vi "Generate Simulated Data.vi"(7 "Type de mode":bool, 8 "error in (no error)":T2 caption="entrée d'erreur (pas d'erreur)", 9 "Péri":tag="Dev1", 10 "Longueur d'onde":dbl, 11 "Type de signal":T1) -> (0 "error out":T2 caption="sortie d'erreur", 2 "Données du graphe":waveform(dbl)[](array[waveform]))   [LabVIEW 2018, in "Acquisition.lvlib"]
doc: "Génère des exemples de waveforms en fonction du type de signal dans l'entrée Configuration du matériel."
uses:
  Acquisition.lvlib
  <vilib>/Analysis/NI_AALBase.lvlib
  Signal Type.ctl
panel:
  out "Graphe déroulant":dynamicdata(graph)
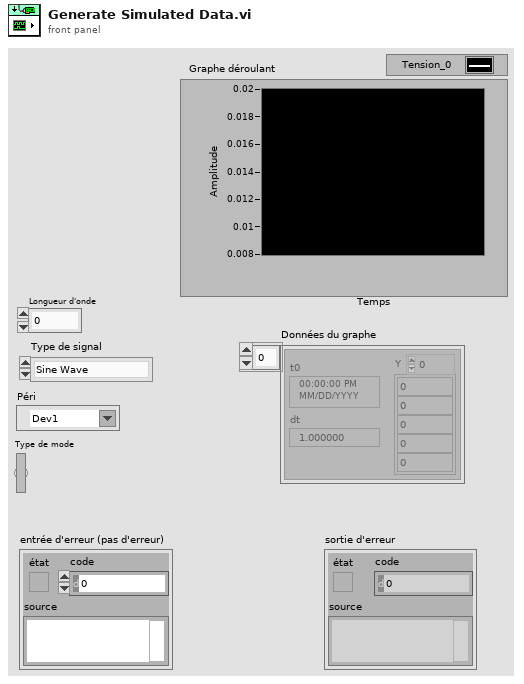
[diagram p1: front panel]
types:
  T1 = typedef "Acquisition.lvlib/Signal Type.ctl" = enum16{"Sine Wave", "Square with Noise", "Signal triangulaire", "Simulation DAQ"}
  T2 = cluster{"état":bool, "code":i32, "source":string}
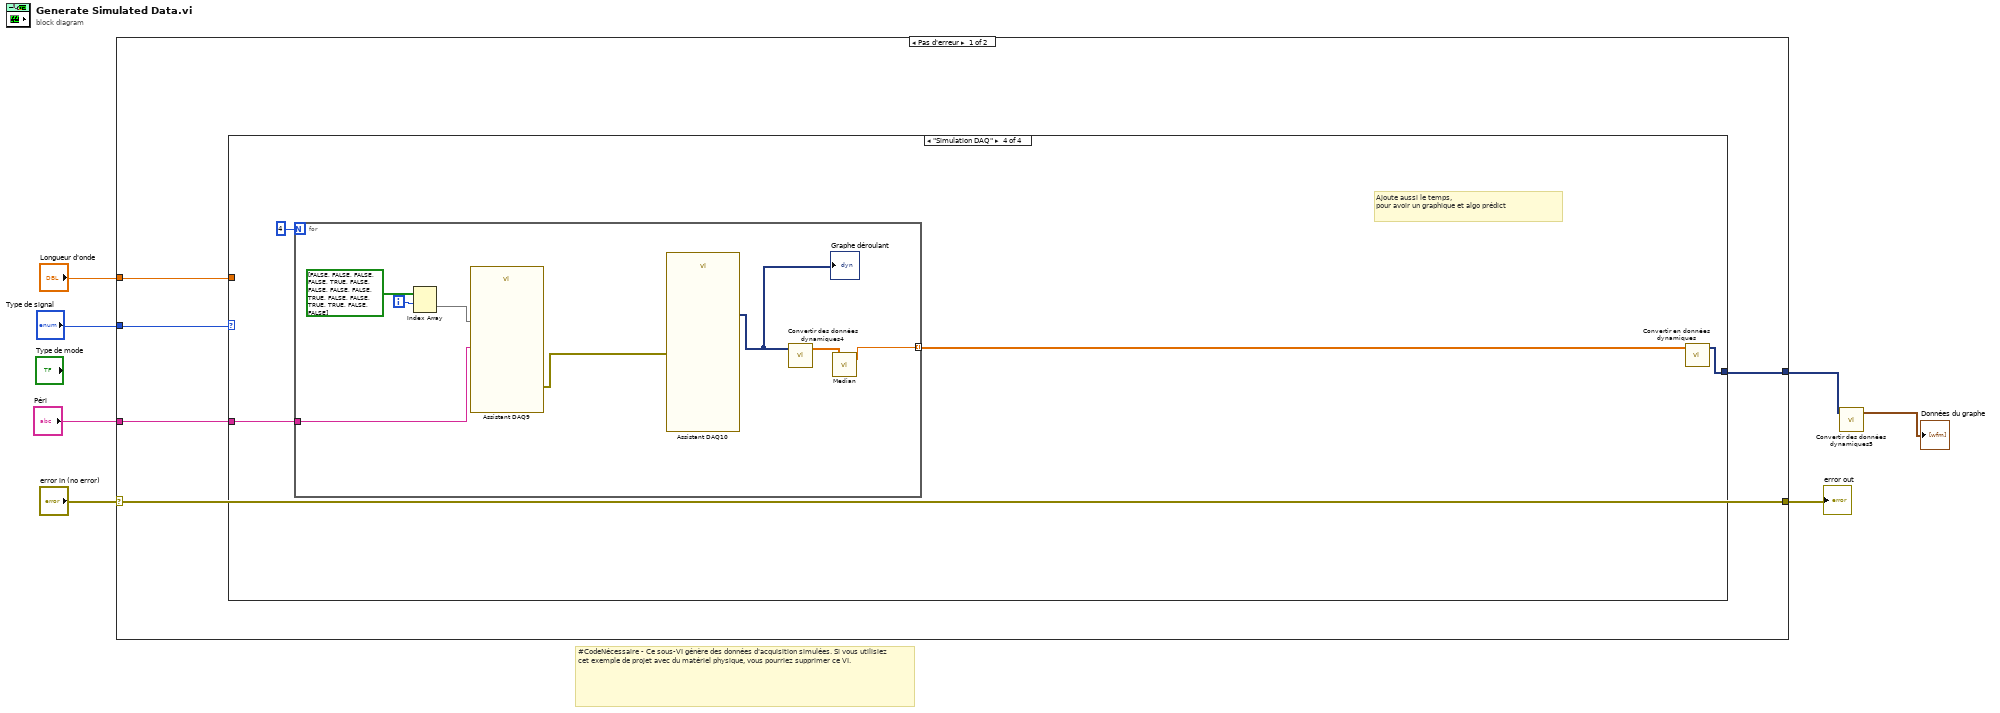
[diagram p0: block diagram]
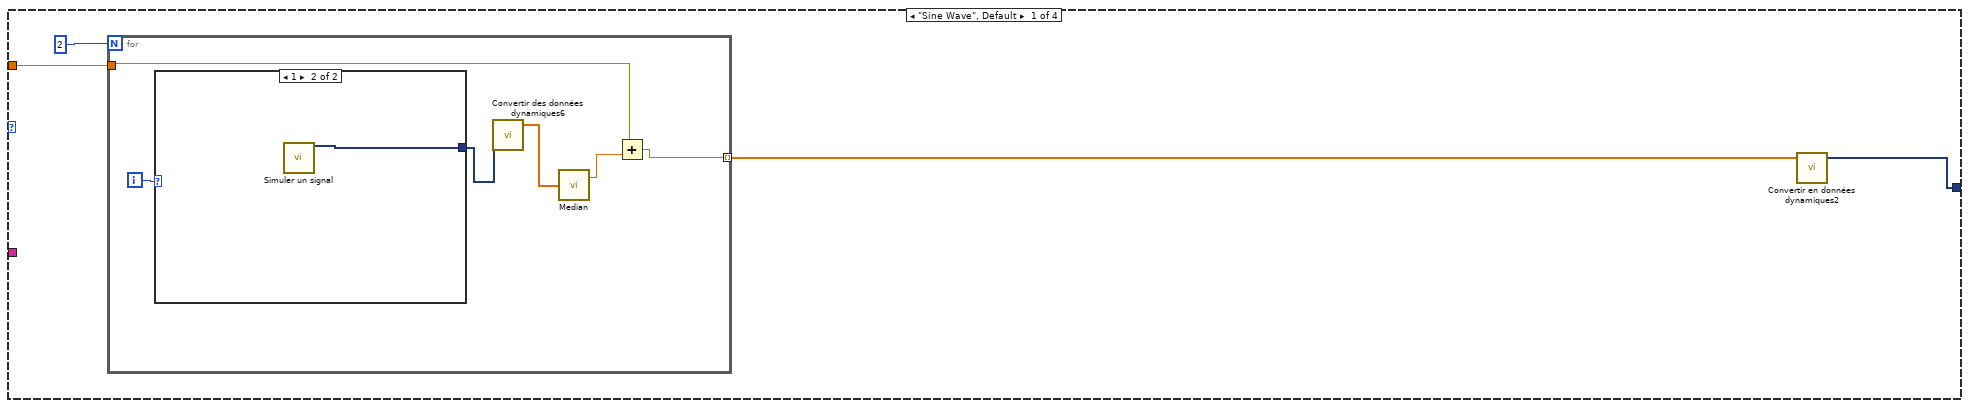
[diagram p2: hidden frame]
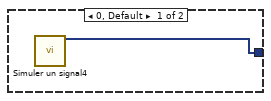
[diagram p3: hidden frame]
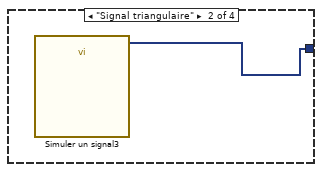
[diagram p4: hidden frame]
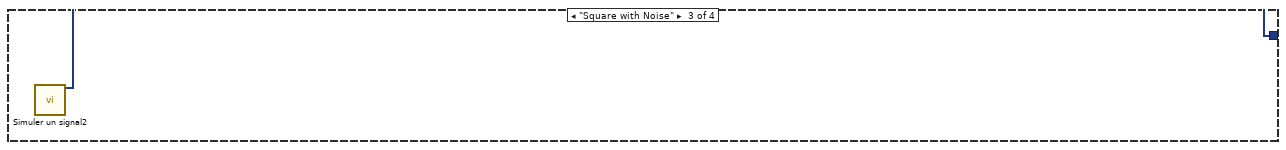
[diagram p5: hidden frame]
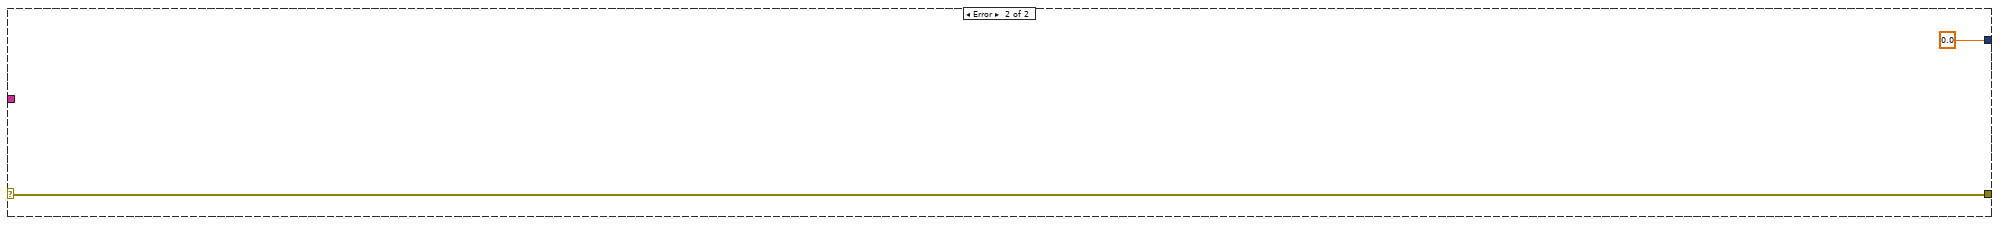
[diagram p6: hidden frame]
diagram:
  # "#CodeNécessaire - Ce sous-VI génère des données d'acquisition simulées. Si vous utilisiez cet exemple de projet avec du matériel physique, vous pourriez supprimer ce VI."
  n1 = case shown="Pas d'erreur" "error in (no error)" {
    selector: "error in (no error)" -> [w12 w40]
    tunnel: [w12 w40] -> w6
    tunnel: "Type de signal" -> [w11 _]
    tunnel: [w10 0.0] -> w3
    tunnel: "Longueur d'onde" -> [w9 _]
    tunnel: "Péri" -> [w8 _]
    frame No Error {
      n2 = case shown="\"Simulation DAQ\"" w11 {
        tunnel: [w15 w25 w26 w29] -> w10
        tunnel: w9 -> [w13 _ _ _]
        tunnel: w8 -> [_ _ _ w27]
        frame "Sine Wave", Default {
          n3 = for {
            N: 2 -> [_]
            tunnel: [w18] -> w14 mode=indexing
            tunnel: w13 -> [w17]
            i -> [w22]
            n4 = case shown="1" w22 {
              tunnel: [w23 w24] -> w21
              frame 0, Default {
                n5 = call "Simuler un signal4"() -> ("CC"=w23:dynamicdata)  [unwired: 14 in, 1 out]
              }
              frame 1 {
                n6 = call "Simuler un signal"() -> ("Sinus avec Bruit uniforme"=w24:dynamicdata)  [unwired: 14 in, 1 out]
              }
            }
            n7 = call "Convertir des données dynamiques6"("Dynamic Data Type"=w21) -> ("Array"=w20:dbl[])  [unwired: 3 in]
            n8 = call <vilib>:"Median.vi"("X"=w20) -> ("median"=w19:dbl)  [unwired: 1 out]
            n9 = Add(x=w17, y=w19) -> (x+y=w18:dbl)
          }
          n10 = call "Convertir en données dynamiques2"("Array"=w14) -> ("Dynamic Data Type"=w15:dynamicdata)  [unwired: 3 in]
        }
        frame "Signal triangulaire" {
          n11 = call "Simuler un signal3"() -> ("Triangle"=w25:dynamicdata)  [unwired: 14 in, 1 out]
        }
        frame "Square with Noise" {
          n12 = call "Simuler un signal2"() -> ("Square with Gaussian Noise"=w26:dynamicdata)  [unwired: 14 in, 1 out]
        }
        frame "Simulation DAQ" {
          # "Ajoute aussi le temps,\npour avoir un graphique et algo prédict"
          n13 = for {
            N: 4 -> [_]
            tunnel: [w38] -> w28 mode=indexing
            tunnel: w27 -> [w31]
            i -> [w33]
            n14 = Index Array(array=bool[][] [[FALSE, FALSE, FALSE, FALSE], [TRUE, FALSE, FALSE, FALSE], [FALSE, TRUE, FALSE, FALSE], [TRUE, TRUE, FALSE, FALSE]], index (row)=w33) -> (element=w32:bool[])  [unwired: 1 in]
            n15 = call "Assistant DAQ9"("data"=w32, "nom du périphérique"=w31) -> ("error out"=w36:errorcluster)  [unwired: 16 in, 1 out]
            n16 = call "Assistant DAQ10"("error in"=w36) -> ("data"=w35:dynamicdata)  [unwired: 16 in, 2 out]
            "Graphe déroulant" <- w35
            n17 = call "Convertir des données dynamiques4"("Dynamic Data Type"=w35) -> ("Array"=w37:dbl[])  [unwired: 3 in]
            n18 = call <vilib>:"Median.vi"("X"=w37) -> ("median"=w38:dbl)  [unwired: 1 out]
          }
          n19 = call "Convertir en données dynamiques"("Array"=w28) -> ("Dynamic Data Type"=w29:dynamicdata)  [unwired: 3 in]
        }
      }
    }
    frame Error {
    }
  }
  "error out" <- w6
  n20 = call "Convertir des données dynamiques5"("Dynamic Data Type"=w3) -> ("Array of Waveform"=→"Données du graphe":waveform(dbl)[])  [unwired: 3 in]
